vi "PRIME Telescope Open TCP Socket.vi"(8 "error in (no error)":errorcluster, 10 "port":u16, 11 "IP Address":string) -> (0 "error out":errorcluster, 3 "connection ID":refnum<k5>)   [LabVIEW 2021, in "PRIME Telescope.lvclass"]
uses:
  PRIME Telescope.lvclass
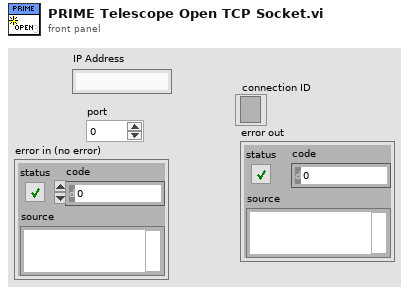
[diagram p1: front panel]
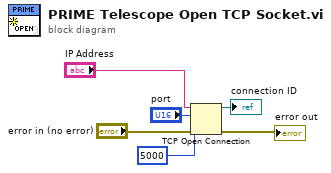
[diagram p0: block diagram]
diagram:
  n1 = TCP Open Connection(address="IP Address", remote port or service name="port", timeout ms (60000)=5000, error in (no error)="error in (no error)") -> (connection ID=→"connection ID":refnum<k5>, error out=→"error out":errorcluster)  [unwired: 1 in]
